vi "Gif.getBlock.vi"(0 "data":u8[](array[numeric]), 9 "offset":i32, 11 "error in (no error)":errorcluster, 12 "label":u8) -> (6 "pos offset":i32, 8 "found?":bool, 10 "offset out":i32, 15 "error out":errorcluster)   [LabVIEW 2019]
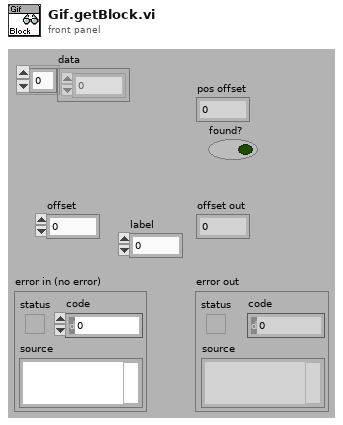
[diagram p1: front panel]
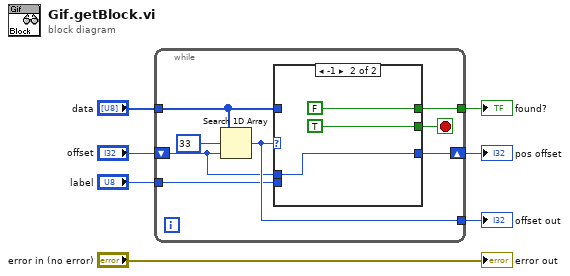
[diagram p0: block diagram]
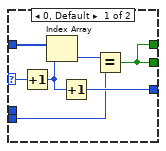
[diagram p2: hidden frame]
diagram:
  n1 = while {
    tunnel: "data" -> [w15]
    shift-right: [w14] -> w4
    shift-left: "offset" -> [w8]
    tunnel: [w12] -> w3
    tunnel: [w10] -> w6
    tunnel: "label" -> [w9]
    stop <- w13 stop-if-true
    n2 = Search 1D Array(1D array=w15, element=u8 33, start index (0)=w8) -> (index of element=w10:i32)
    n3 = case shown="-1" w10 {
      selector: w10 -> [w17 _]
      tunnel: w15 -> [w22 _]
      tunnel: [w20 w23] -> w14
      tunnel: [w18 TRUE] -> w13
      tunnel: [w18 FALSE] -> w12
      tunnel: w9 -> [w16 _]
      tunnel: w8 -> [_ w23]
      frame 0, Default {
        n4 = Increment(x=w17) -> (x+1=w21:i32)
        n5 = Index Array(array=w22, index=w21) -> (element=w19:u8)
        n6 = Increment(x=w21) -> (x+1=w20:i32)
        n7 = Equal?(x=w19, y=w16) -> (x = y?=w18:bool)
      }
      frame -1 {
      }
    }
  }
  "offset out" <- w6
  "pos offset" <- w4
  "found?" <- w3
  "error out" <- "error in (no error)"
